vi "timing_data_to_boolean_array.vi"(2 "end time [us]":dbl=1.0, 3 "start time [us]":dbl, 4 "overall length [us]":dbl=1000.0) -> (0 "boolean timing array":bool[](array[boolean]))   [LabVIEW 2011]
doc: "Creates a boolean array based on the timing info send in. Used to display a digital waveform graph to visualize the timing info recieved and send to the Standford Research Systems DG645 Delay Generator."
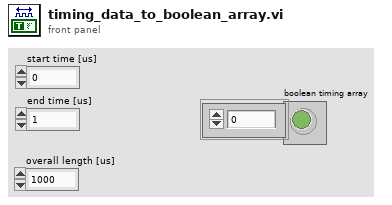
[diagram p1: front panel]
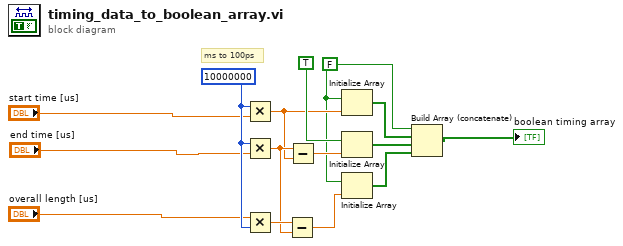
[diagram p0: block diagram]
diagram:
  w5 = FALSE
  w15 = 10000000 ("y")
  # "ms to 100ps"
  n1 = Multiply(x=w15, y="start time [us]") -> (x*y=w7:dbl)
  n2 = Multiply(x=w15, y="end time [us]") -> (x*y=w8:dbl)
  n3 = Multiply(x="overall length [us]", y=w15) -> (x*y=w13:dbl)
  n4 = Subtract(x=w13, y=w8) -> (x-y=w12:dbl)
  n5 = Subtract(x=w8, y=w7) -> (x-y=w6:dbl)
  n6 = Initialize Array(w5, w7) -> (w14:bool[])
  n7 = Initialize Array(TRUE, w6) -> (w9:bool[])
  n8 = Initialize Array(w5, w12) -> (w11:bool[])
  n9 = Build Array (concatenate)(w5, w14, w9, w11) -> (→"boolean timing array":bool[])
